vi "get aliases and matching dev var name.vi"() -> (2 "dev name \"space\" var name":string[](array[string]), 3 "alias":string[](array[string]))   [LabVIEW 2020]
uses:
  MySQL/Preset Query Enum.ctl
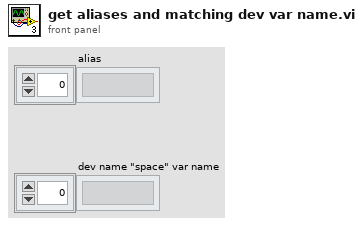
[diagram p1: front panel]
types:
  T1 = typedef "Preset Query Enum.ctl" = enum16{"Get Locations", "Get all IPs and MACs", "Get classes", "Get expt variables to set at scanstart for particular device", "Get expt devices and variables with start values", "Get expt devices and variables (with data to get)", "Get expt devices with data to get", "Get Expt devices and GUIs", "Get all devices basic properties", "Get Virtual Devices Core Info", "Get Expt names", "Get experiment basic properties", "Get experiment alarm variables", "Get MC Ports", "Get device network comm port", "Get devicetype lvclass path", "Get basic device properties", "Get Init Order", "Get all setable variables of a device", "Get device variable aliases", "Get force values of all settable variables", "Get all variables of a devicetype", "Get all variables of a device", "Get plotter details", "Get Saved Scans", "Get Scan Info", "GetGeneralGUIs", "Get expt for plotter", "Get plotter IDs from expt", "Get all devices", "Get all Virtual Devices", "Get all aliases", "Get variable and device info for Virtual Device", "GetItemLocatorIP", "Get IPs for GUIs", "Get DeviceType from Device", "GetLocalPortRange", "GetDevicePresetVariables", "Get Device Configuration", "GetAllPresetNames", "GetAllConfigurationNames", "GetPresetDeviceNames", "GetDeviceAliases", "GetDevicesOfClass"}
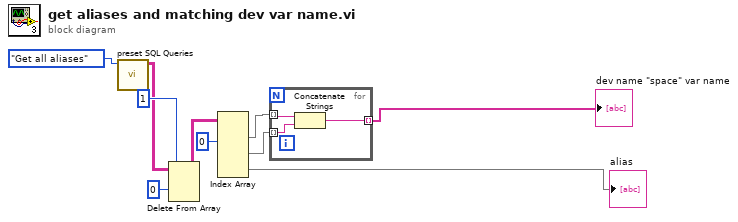
[diagram p0: block diagram]
diagram:
  n1 = call "preset SQL Queries.vi"("Preset Query"=Preset_Query_Enum."Get all aliases") -> ("data"=w2:string[][])  [unwired: 8 in, 2 out]
  n2 = Delete From Array(array=w2, length=1, index (row)=0) -> (array with subset deleted=w5:string[][])  [unwired: 1 in, 1 out]
  n3 = Index Array(array=w5, index (col) #1=0 ("disabled index (col)")) -> (element #1=w8:string[], element #2=w9:string[], element #3=→"alias":string[])  [unwired: 5 in]
  n4 = for {
    tunnel: w8 -> [w13] mode=indexing
    tunnel: w9 -> [w12] mode=indexing
    tunnel: [w11] -> w10 mode=indexing
    n5 = Concatenate Strings(w13, w12) -> (w11:string)
  }
  "dev name \"space\" var name" <- w10
